vi "Reformat Target.vi"(8 "error in (no error)":errorcluster, 10 "IP Address":string, 11 "Ctl Refs in":T1) -> (0 "error out":errorcluster, 3 "Ctl Refs out":T1)   [LabVIEW 2013]
uses:
  Controls/Refs.ctl
  Controls/Button Refs.ctl
  Controls/Tab Ctl Refs.ctl
  types/TabStateType.ctl
  Controls/Indicator Refs.ctl
  Controls/Slider Refs.ctl
  Controls/Control Refs.ctl
  <vilib>/nisyscfg/Initialize (String).vi
  <vilib>/nisyscfg/Close (System).vi
  <vilib>/nisyscfg/nisyscfg.lvlib
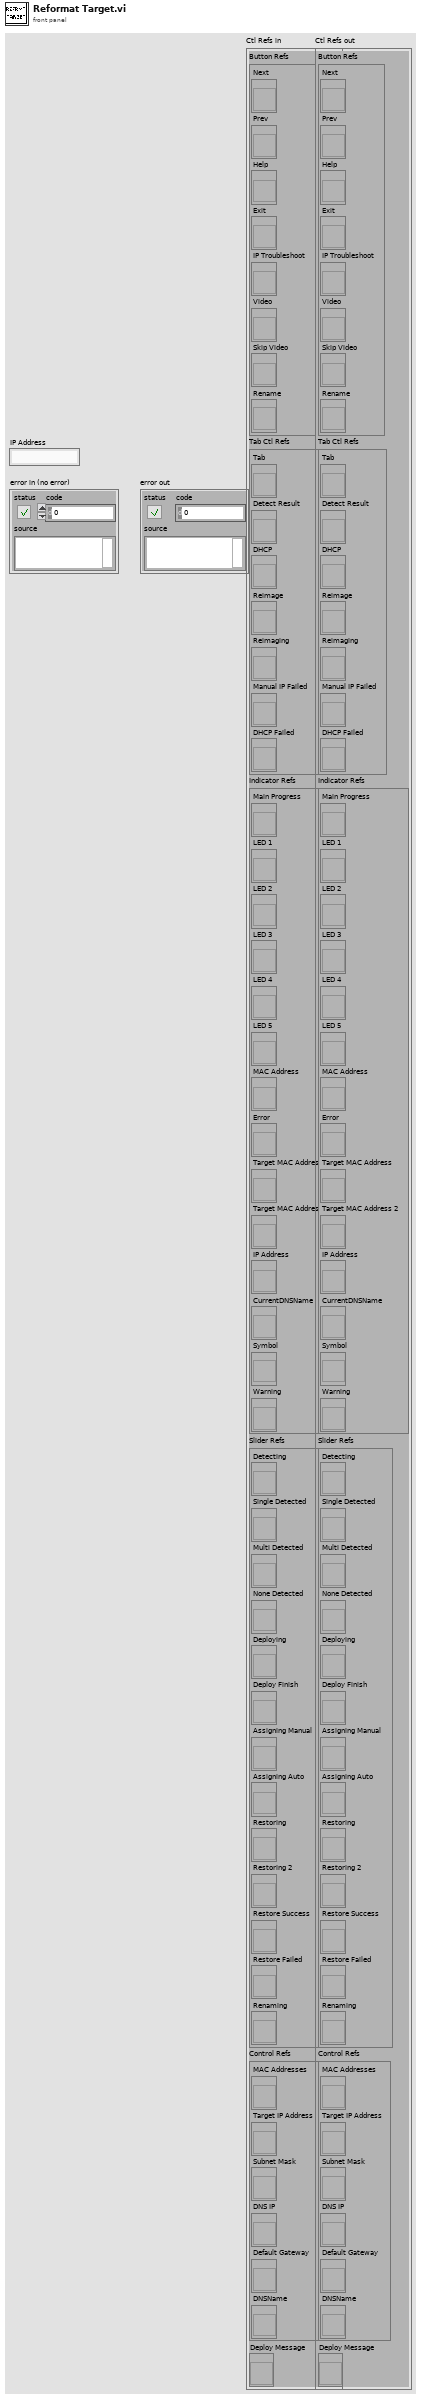
[diagram p1: front panel]
types:
  T1 = typedef "Refs.ctl" = cluster{"Button Refs":T2, "Tab Ctl Refs":T3, "Indicator Refs":T4, "Slider Refs":T5, "Control Refs":T6, "Deploy Message":refnum<vi>}
  T2 = typedef "Button Refs.ctl" = cluster{"Next":refnum<vi>, "Prev":refnum<vi>, "Help":refnum<vi>, "Exit":refnum<vi>, "IP Troubleshoot":refnum<vi>, "Video":refnum<vi>, "Skip Video":refnum<vi>, "Rename":refnum<vi>}
  T3 = typedef "Tab Ctl Refs.ctl" = cluster{"Tab":refnum<vi>, "Detect Result":refnum<vi>, "DHCP":refnum<vi>, "Reimage":refnum<vi>, "Reimaging":refnum<vi>, "Manual IP Failed":refnum<vi>, "DHCP Failed":refnum<vi>}
  T4 = typedef "Indicator Refs.ctl" = cluster{"Main Progress":refnum<vi>, "LED 1":refnum<vi>, "LED 2":refnum<vi>, "LED 3":refnum<vi>, "LED 4":refnum<vi>, "LED 5":refnum<vi>, "MAC Address":refnum<vi>, "Error":refnum<vi>, "Target MAC Address":refnum<vi>, "Target MAC Address 2":refnum<vi>, "IP Address":refnum<vi>, "CurrentDNSName":refnum<vi>, "Symbol":refnum<vi>, "Warning":refnum<vi>}
  T5 = typedef "Slider Refs.ctl" = cluster{"Detecting":refnum<vi>, "Single Detected":refnum<vi>, "Multi Detected":refnum<vi>, "None Detected":refnum<vi>, "Deploying":refnum<vi>, "Deploy Finish":refnum<vi>, "Assigning Manual":refnum<vi>, "Assigning Auto":refnum<vi>, "Restoring":refnum<vi>, "Restoring 2":refnum<vi>, "Restore Success":refnum<vi>, "Restore Failed":refnum<vi>, "Renaming":refnum<vi>}
  T6 = typedef "Control Refs.ctl" = cluster{"MAC Addresses":refnum<vi>, "Target IP Address":refnum<vi>, "Subnet Mask":refnum<vi>, "DNS IP":refnum<vi>, "Default Gateway":refnum<vi>, "DNSName":refnum<vi>}
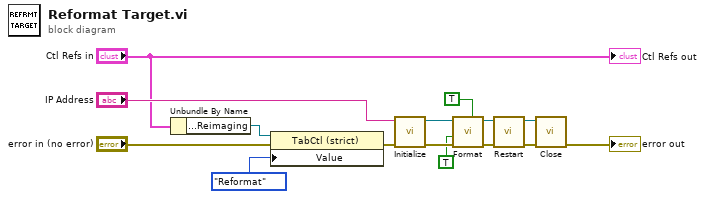
[diagram p0: block diagram]
diagram:
  n1 = Unbundle By Name("Ctl Refs in") -> ("Tab Ctl Refs.Reimaging"=w9:refnum<vi>)
  n2 = property on="Property Node" class="TabCtl (strict)"(reference=w9, error in="error in (no error)", "Value"=enum32{"Reformat", "Reimage", "IP Config"}."Reformat" ("Reimaging Tabs")) -> (error out=w11:errorcluster)  [unwired: 1 out]
  n3 = call-poly <vilib>:"Initialize.vi"("error in (no error)"=w11, "target (localhost)"="IP Address") -> ("error out"=w14:errorcluster, "session out"=w13:refnum<k21>)  [unwired: 7 in, 1 out]
  n4 = call <vilib>:"Format.vi"("force safe mode (F)"=TRUE, "error in (no error)"=w14, "keep network settings (F)"=TRUE, "session in"=w13) -> ("error out"=w6:errorcluster, "session out"=w2:refnum<k21>)  [unwired: 6 in]
  n5 = call <vilib>:"Restart.vi"("error in (no error)"=w6, "session in"=w2) -> ("error out"=w3:errorcluster, "session out"=w1:refnum<k21>)  [unwired: 7 in, 1 out]
  n6 = call-poly <vilib>:"Close.vi"("error in (no error)"=w3, "session in"=w1) -> ("error out"=→"error out":errorcluster)  [unwired: 9 in]
  "Ctl Refs out" <- "Ctl Refs in"
